vi "Query Port Resources.vi"(8 "error in (no error)":errorcluster, 10 "port":u32, 11 "board":u32) -> (0 "error out":errorcluster, 1 "found":bool, 3 "port resource":T1)   [LabVIEW 2020, in "AIM664LV.lvlib"]
uses:
  AIM664LV.lvlib
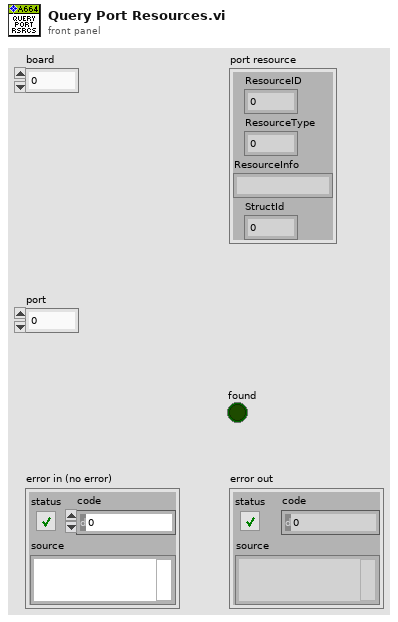
[diagram p1: front panel]
types:
  T1 = cluster{"ResourceID":u32, "ResourceType":u32, "ResourceInfo":string, "StructId":u32}
  T2 = typedef "AIM664LV.lvlib/hwResource_port.ctl" = cluster{"boardId":u32, "portId":u32, "ServerResourceInfo":cluster{"ResourceID":u32, "ResourceType":u32, "ResourceInfo":string, "StructId":u32}}
  T3 = typedef "AIM664LV.lvlib/hwResource_board.ctl" = cluster{"boardId":u32, "ServerResourceInfo":cluster{"ResourceID":u32, "ResourceType":u32, "ResourceInfo":string, "StructId":u32}}
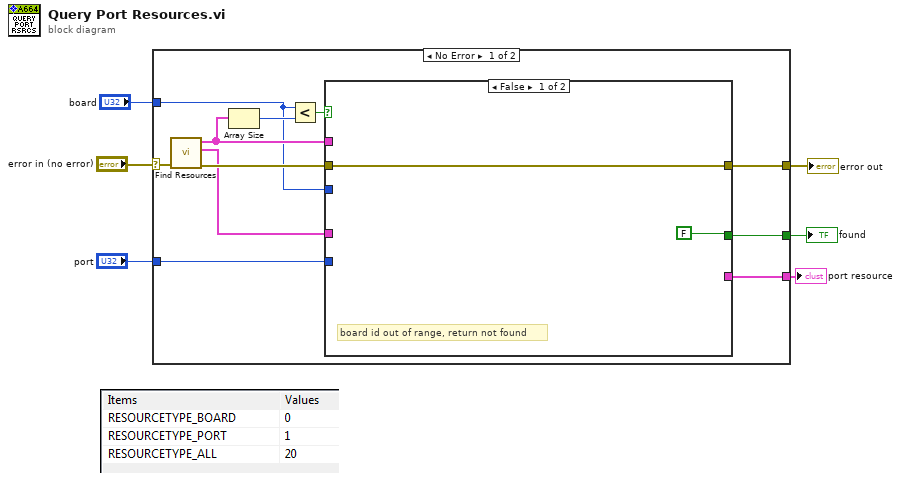
[diagram p0: block diagram]
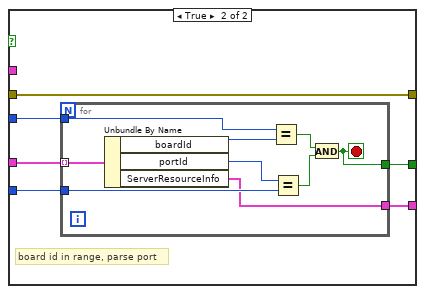
[diagram p2: hidden frame]
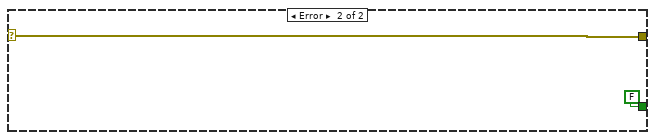
[diagram p3: hidden frame]
diagram:
  n1 = case shown="No Error" "error in (no error)" {
    selector: "error in (no error)" -> [w17 w36]
    tunnel: "port" -> [w14 _]
    tunnel: "board" -> [w11 _]
    tunnel: [w8 w36] -> w3
    tunnel: [w9 _] -> w2
    tunnel: [w7 FALSE ("found")] -> w1
    frame No Error {
      n2 = call "Find Resources.vi"("error in"=w17) -> ("error out"=w15:errorcluster, "Ports"=w10:T2[], "Boards"=w13:T3[])  [unwired: 8 in]
      n3 = Array Size(array=w13) -> (size(s)=w12:i32)
      n4 = Less?(x=w11, y=w12) -> (x < y?=w16:bool)
      n5 = case shown="False" w16 {
        tunnel: w15 -> [w18 w24]
        tunnel: w14 -> [_ w22]
        tunnel: w13 -> [_ _]
        tunnel: w11 -> [_ w23]
        tunnel: w10 -> [_ w25]
        tunnel: [_ w20] -> w9
        tunnel: [w18 w24] -> w8
        tunnel: [FALSE w21] -> w7
        frame False {
          # "board id out of range, return not found"
        }
        frame True {
          # "board id in range, parse port"
          n6 = for {
            tunnel: w25 -> [w34] mode=indexing
            tunnel: w23 -> [w30]
            tunnel: w22 -> [w31]
            tunnel: [w27] -> w20
            tunnel: [w26] -> w21
            stop <- w26 stop-if-true
            n7 = Unbundle By Name(w34) -> ("boardId"=w33:u32, "portId"=w32:u32, "ServerResourceInfo"=w27:T1)
            n8 = Equal?(x=w30, y=w33) -> (x = y?=w29:bool)
            n9 = Equal?(x=w32, y=w31) -> (x = y?=w28:bool)
            n10 = And(x=w29, y=w28) -> (x .and. y?=w26:bool)
          }
        }
      }
    }
    frame Error {
    }
  }
  "error out" <- w3
  "port resource" <- w2
  "found" <- w1
